vi "Read Transfer Settings ID.vi"(8 "error in (no error)":errorcluster, 10 "Transfer ID":string, 11 "Configuration Session in":refnum<class "Configuration Session.lvclass">) -> (0 "error out":errorcluster, 1 "Settings ID":string, 3 "Configuration Session out":refnum<class "Configuration Session.lvclass">, 4 "found?":bool)   [LabVIEW 2017, in "DSF Core.lvlib" / "Configuration Session.lvclass"]
uses:
  Configuration Session.lvclass
  Configuration Session.lvclass/Configuration Session.ctl
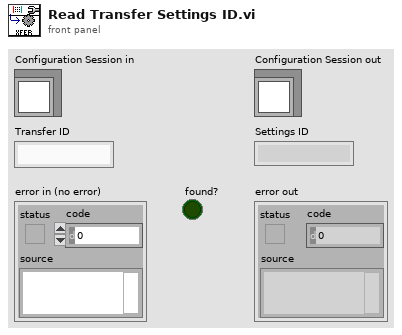
[diagram p1: front panel]
types:
  T1 = typedef "DSF Core.lvlib/Configuration Session.lvclass/DSF Config Data Ref.ctl" = refnum<data-value>
  T2 = typedef "DSF Core.lvlib/Configuration Session.lvclass/DSF Config Data.ctl" = cluster{"dsf configuration":T3, "path":path, "dirty":bool}
  T3 = typedef "DSF Core.lvlib/Configuration Session.lvclass/Internal DSF Configuration.ctl" = cluster{"dsfversion":T4, "version":T4, "plugins":T5[], "groups":T10[], "transfers":T12[], "channels":T14[], "settings":T16[]}
  T4 = typedef "DSF Core.lvlib/DSF Version Info.ctl" = cluster{"major":u32, "minor":u32, "fix":u32, "build":string}
  T5 = typedef "DSF Core.lvlib/Configuration Session.lvclass/Internal DSF Plugin with ID.ctl" = cluster{"id":string, "values":T6}
  T6 = typedef "DSF Core.lvlib/Configuration Session.lvclass/Internal DSF Plugin Info.ctl" = cluster{"components":string[], "timing":T7, "group ids":string[], "settings id":string, "threads":T8[]}
  T7 = typedef "DSF Core.lvlib/DSF Timing Info.ctl" = cluster{"priority":u64, "decimation":u64, "offset":u64}
  T8 = typedef "DSF Core.lvlib/DSF Engine Plugin Thread Configuration.ctl" = cluster{"buffer converter settings":T9, "transceiver settings":T9, "custom settings":T9, "processor":i32, "priority offset":i16}
  T9 = typedef "DSF Core.lvlib/DSF Settings Info.ctl" = cluster{"key":string, "value":string}[]
  T10 = typedef "DSF Core.lvlib/Configuration Session.lvclass/Internal DSF Group with ID.ctl" = cluster{"id":string, "values":T11}
  T11 = typedef "DSF Core.lvlib/Configuration Session.lvclass/Internal DSF Group Info.ctl" = cluster{"direction":i32, "timing":T7, "transfer ids":string[], "settings id":string, "thread":i32, "timeout behavior":u8}
  T12 = typedef "DSF Core.lvlib/Configuration Session.lvclass/Internal DSF Transfer with ID.ctl" = cluster{"id":string, "values":T13}
  T13 = typedef "DSF Core.lvlib/Configuration Session.lvclass/Internal DSF Transfer Info.ctl" = cluster{"byte order":i32, "channel ids":string[], "settings id":string}
  T14 = typedef "DSF Core.lvlib/Configuration Session.lvclass/Internal DSF Channel with ID.ctl" = cluster{"id":string, "values":T15}
  T15 = typedef "DSF Core.lvlib/Configuration Session.lvclass/Internal DSF Channel Info.ctl" = cluster{"string buffer offset":u64, "string data type":i32, "engine data type":i32, "settings id":string, "units":string}
  T16 = typedef "DSF Core.lvlib/Configuration Session.lvclass/Internal DSF Settings with ID.ctl" = cluster{"id":string, "values":T17}
  T17 = typedef "DSF Core.lvlib/Configuration Session.lvclass/Internal DSF Settings Info.ctl" = cluster{"key":string, "value":string}[]
  T18 = typedef "DSF Core.lvlib/DSF Group Info.ctl" = cluster{"direction":T19, "timing":T7, "transfer ids":string[], "settings id":string, "thread":i32, "timeout behavior":T20}
  T19 = typedef "DSF Core.lvlib/DSF Direction.ctl" = enum8{"Tx", "Rx"}
  T20 = typedef "DSF Core.lvlib/DSF Timeout Behavior.ctl" = enum8{"Increment Late Count", "Throw Error"}
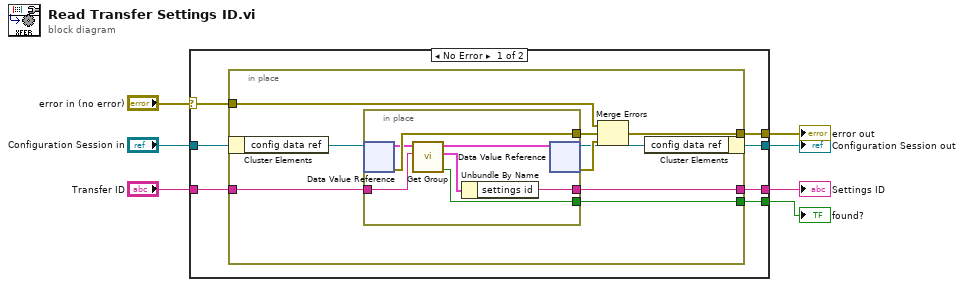
[diagram p0: block diagram]
diagram:
  n1 = case shown="No Error" "error in (no error)" {
    selector: "error in (no error)" -> [w14 w32]
    tunnel: "Configuration Session in" -> [w9 w31]
    tunnel: [w12 w32] -> w5
    tunnel: "Transfer ID" -> [w13 _]
    tunnel: [w11 _] -> w3
    tunnel: [w10 _] -> w2
    tunnel: [w8 w31] -> w1
    frame No Error {
      n2 = in-place {
        in-place-border: w14 -> [w23]
        in-place-border: w13 -> [w22]
        in-place-border: [w21] -> w12
        in-place-border: [w18] -> w11
        in-place-border: [w17] -> w10
        n3 = in-place-cluster #1(w9) -> ("config data ref"=w16:T1)
        n4 = in-place {
          in-place-border: w22 -> [w28]
          in-place-border: [w30] -> w20
          in-place-border: [w27] -> w18
          in-place-border: [w24] -> w17
          n5 = in-place-dvr #2(w16) -> (w29:T2, w30:errorcluster)
          n6 = call "Get Group.vi"("id"=w28, "DSF Configuration in"=w29) -> ("exists?"=w27:bool, "info"=w25:T18, "DSF Configuration out"=w26:T2)  [unwired: 6 in, 1 out]
          n7 = Unbundle By Name(w25) -> ("settings id"=w24:string)
          n8 = in-place-dvr #2(w26) -> (w15:T1, w19:errorcluster)
        }
        n9 = Merge Errors(w23, w20, w19) -> (w21:errorcluster)
        n10 = in-place-cluster #1("config data ref"=w15) -> (w8:refnum<class "Configuration Session.lvclass">)
      }
    }
    frame Error {
    }
  }
  "error out" <- w5
  "found?" <- w3
  "Configuration Session out" <- w1
  "Settings ID" <- w2
